vi "Log Message.vi"(8 "error in (no error)":errorcluster, 10 "String":string, 11 "Log in":refnum<class "Log.lvclass">) -> (0 "error out":errorcluster, 3 "Log out":refnum<class "Log.lvclass">)   [LabVIEW 2015, in "AMS UI.lvlib" / "Log.lvclass"]
uses:
  Log.lvclass
  Log.lvclass/Log.ctl
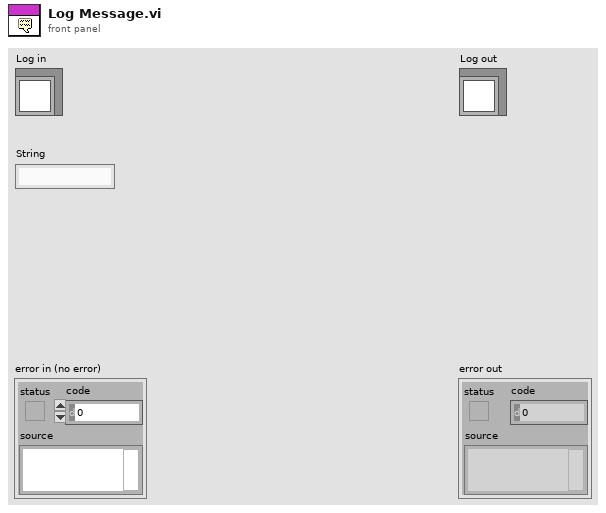
[diagram p1: front panel]
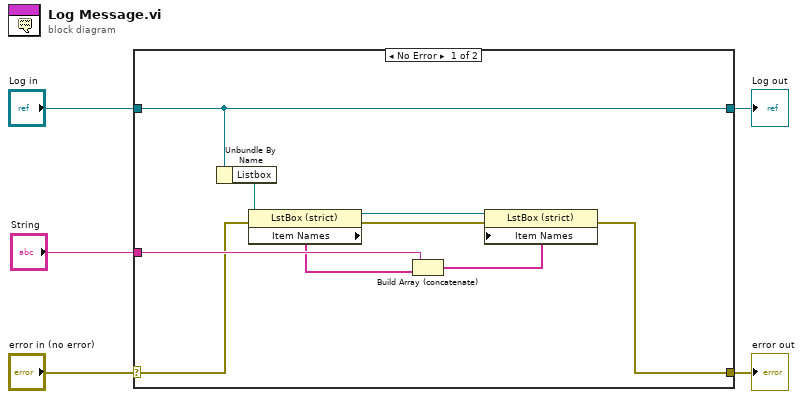
[diagram p0: block diagram]
diagram:
  n1 = case shown="No Error" "error in (no error)" {
    selector: "error in (no error)" -> [w7 w16]
    tunnel: [w6 w16] -> w4
    tunnel: [w14 w15] -> w2
    tunnel: "Log in" -> [w14 w15]
    tunnel: "String" -> [w12 _]
    frame No Error {
      n2 = Unbundle By Name(w14) -> ("Listbox"=w13:refnum<vi>)
      n3 = property class="LstBox (strict)"(reference=w13, error in=w7) -> (reference out=w10:refnum<vi>, error out=w11:errorcluster, "Item Names"=w9:string[])
      n4 = Build Array (concatenate)(w12, w9) -> (w8:string[])
      n5 = property class="LstBox (strict)"(reference=w10, error in=w11, "Item Names"=w8) -> (error out=w6:errorcluster)  [unwired: 1 out]
    }
    frame Error {
    }
  }
  "error out" <- w4
  "Log out" <- w2
